vi "Filter out non-nummeric characters.vi"(2 "string in":string) -> (6 "string out":string)   [LabVIEW 2015, in "Powermeter_library.lvlib"]
uses:
  Powermeter_library.lvlib
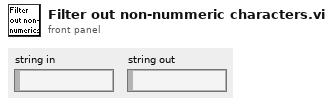
[diagram p1: front panel]
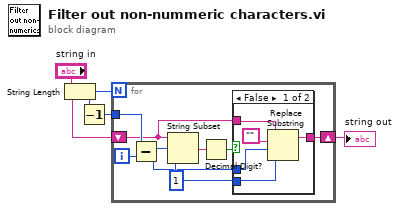
[diagram p0: block diagram]
diagram:
  n1 = String Length(string="string in") -> (length=w3:i32)
  n2 = Decrement(x=w3) -> (x-1=w2:i32)
  n3 = for {
    N: w3 -> [_]
    shift-right: [w8] -> w1
    shift-left: "string in" -> [w7]
    tunnel: w2 -> [w11]
    i -> [w10]
    w6 = 1 ("length (rest)")
    n4 = Subtract(x=w11, y=w10) -> (x-y=w5:i32)
    n5 = String Subset(string=w7, offset (0)=w5, length (rest)=w6) -> (substring=w12:string)
    n6 = Decimal Digit?(1:w12) -> (0:w9:bool)
    n7 = case shown="False" w9 {
      tunnel: [w16 w18] -> w8
      tunnel: w7 -> [w17 w18]
      tunnel: w6 -> [w15 _]
      tunnel: w5 -> [w14 _]
      frame False {
        n8 = Replace Substring(2:w15, 3:w14, 4:"", 5:w17) -> (1:w16:string)  [unwired: 1 out]
      }
      frame True {
      }
    }
  }
  "string out" <- w1
